vi "DOE Auto Rinse Detect.vi"(9 "Condition Name In Column":string="RINSE", 10 "Column Name":string="Sub-Cycle", 11 "GEA Input Data":string[][](array[string])=[["System Time", "18:08.8"], ["Elapsed Time", "19379.67345"], ["Cold Water Temperature (F)", "55.796"], ["Hot Water Temperature (F)", "134.611"], ["Cold Water Pressure (PSI)", "35.043"], ["Hot Water Pressure (PSI)", "34.892"], ["Ambient Temperature (F)", "66.383"], ["Room Humidity (%RH)", "55.342"], ["Scale Weight (lbs)", "0.038"], ["Hot Water Total (Gallons)", "2.04"], ["Cold Water Total (Gallons)", "13.53"], ["Hot Water Rate (GPM)", "0"], ["Cold Water Rate (GPM)", "0"], ["Cold Water Total During Wash (Gallons)", "9.61"], ["Hot Water Total During Wash (Gallons)", "2.04"], ["Cold Water Total During Rinse (Gallons)", "3.92"], ["Hot Water Total During Rinse (Gallons)", "0"], ["Voltage (V)", "120.6"], ["RMS Current (Amps)", "0.058"], ["Power (Watts)", "1.534"], ["Watt Hours (Wh)", "105.76"], ["Voltage Total Harmonic Distortion", "0.076"], ["Frequency (Hz)", "59.963"], ["Apparent Power (VA)", "7.044"], ["Power Factor", "0.218"], ["Current Crest Factor", "6.307"], ["Voltage Crest Factor", "1.417"], ["Integration Time (sec)", "2340"], ["Date", "8/26/2016"], ["Time", "15:18:06:.789"], ["APP Version", "Crit 1.10 Non Crit 3.5"], ["XML Version", "Crit 3.5 Non Crit 4.0"], ["Daily Build", "773"], ["Machine State", "IDLE"], ["Motor Profile", "0"], ["Motor Profile Status", "Stopped"], ["Motor Mode", "Idle"], ["Cycle Selected", "Cycle 0"], ["Cycle Engine Status", "Cycle 0 Stopped"], ["Temperature (F)", "74"], ["Lid Status", "Lid Closed"], ["Basket Speed (RPM)", "0"], ["Motor Current RMS (AMPS)", "0.07"], ["Tub Volume (Gal)", "0"], ["Pressure (in H2O)", "0"], ["Lid Lock Status", "Unlocked"], ["Mode Shift Status", "Spin State"], ["Hot Water Valve", "OFF"], ["Cold Water Valve", "OFF"], ["Spray/Rinse Valve", "OFF"], ["Fabric Softener Valve", "OFF"], ["Drain Pump", "OFF"], ["Recirculation Pump", "OFF"], ["Sub-Cycle", "RINSE"], ["Cycle Count", "6"], ["Shaft Speed", "0"], ["ME Relay", "OFF"], ["Valve Relay", "OFF"], ["MS Motor", "OFF"], ["Deep Fill", "OFF"], ["Warm Rinse", "OFF"], ["Deep Rinse/FS", "OFF"], ["My Cycle", "OFF"], ["Extra Rinse", "OFF"], ["Temp Level", "COLORS"], ["Soil Level", "NORMAL"], ["Spin Level", "NORMAL"], ["Load Size", "PRECISE FILL"], ["Stain", "OFF"], ["Delay Time", "0"], ["Soak Time", "0"], ["Auto Soak Level", "0"], ["Dry Load Size", "2047.97"], ["Wet Load Gallons", "4.39"], ["Target Gallons", "4"], ["Load Type", "UNKNOWN"], ["Target Level (inches)", "0"], ["Mode Shift Feedback", "LOW"], ["Red. Version", "5"], ["Red. Pressure", "0.03"], ["Red. Shaft Speed", "0"], ["Red. Mode Shift FB", "00 - Agitate"], ["Red. Lid Switch", "1"], ["Red. Lid Lock", "0"], ["Red. Motor Enable", "1"], ["Red. Triac Enable", "1"], ["Red. Drain Pump", "0"], ["Red. Lid Lock  Speed Interlock", "0"], ["Red. Flood State", "0"], ["Red. Lid Open  Fault State", "0"], ["Red. Unlock Fault State", "0"], ["Red. Access to Moving Parts", "0"], ["Redundant Heartbeat", "0"], ["Segment Gallons", "0"], ["Target Bath Temp (F)", "70"], ["Current Bath Temp (F)", "69.8"], ["ERD 1", "121.84"], ["ERD 2", "121.84"], ["ERD 3", "121.84"], ["Lid Lock FB", "UNLOCKED"], ["Hot Gallons", "0"], ["Cold Gallons", "0"], ["Hot Inlet Temp", "133.7"], ["Cold Inlet temp", "57.3"], ["Warm Inlet Temp", "0"], ["Hot Seg Valve Time", "6"], ["Cold Seg Valve Time", "29"], ["Coast Time", "23736"], ["Ramp Time", "3118"], ["Ramp Speed", "104"], ["Ramp Avg Current", "11.04"], ["Partial Coast Time", "15973"], ["Dry Load Size", "2047.97"], ["Ramp Line Voltage", "115.41"], ["Coast Line Voltage", "120.37"], ["Lid Lock Req State", "UNLOCKED"], ["OOB Det in Accel", "0"], ["Folding in Accel", "2820"], ["Max Jerk in Accel", "36300"], ["OOB det in S-S", "0"], ["Max Jerk in S-S", "0"], ["OOB Redist Req", "0"], ["Remaining Cycle Time (s)", "2280"], ["Available Free Stack %", "49"], ["Child Safety", "OFF"], ["Target Speed", "0"], ["Fault 0", "Reset Clear (1)"], ["Fault 1", ""], ["Fault 2", ""], ["Fault 3", ""], ["Fault 4", ""], ["Fault 5", ""], ["Fault 6", ""], ["Fault 7", ""], ["Fault 8", ""], ["Fault 9", ""], ["Personality", "3"], ["Reset Source", "00 00 0"]]) -> (3 "Condition Found?":bool)   [LabVIEW 2016]
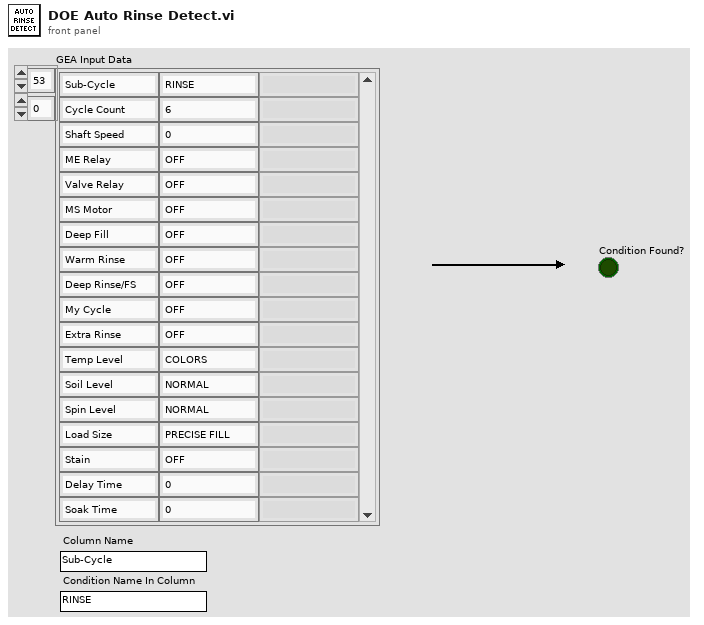
[diagram p1: front panel]
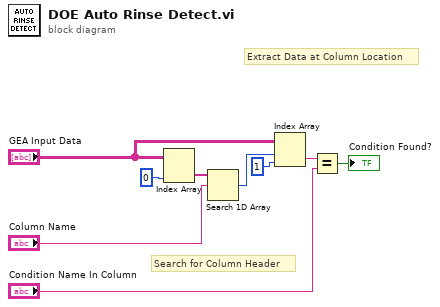
[diagram p0: block diagram]
diagram:
  # "Extract Data at Column Location"
  # "Search for Column Header"
  n1 = Index Array(array="GEA Input Data", index (col)=0 ("disabled index (col)")) -> (element=w8:string[])  [unwired: 1 in]
  n2 = Search 1D Array(1D array=w8, element="Column Name") -> (index of element=w4:i32)  [unwired: 1 in]
  n3 = Index Array(array="GEA Input Data", index (row)=w4, index (col)=1 ("disabled index (col)")) -> (element=w3:string)
  n4 = Equal?(x=w3, y="Condition Name In Column") -> (x = y?=→"Condition Found?":bool)
